vi "Adam_Ch_Input_Output_ASYNC.vi"(4 "Client Name":string, 6 "Previous Scan Value":dbl format="%.2f", 7 "Value to Output":dbl format="%.2f", 8 "Ch values":dbl[](array[numeric]) format="%.2f", 9 "Scan Period":dbl format="%.2f", 10 "Ch Description":T1={"Ch Name"="", "Type"="", "Function"=enum."Analogue Input", "Ch State"=enum."On", "Calibration type"="", "A"=0.0, "B"=0.0, "C"=0.0, "D"=0.0, "Comments"="", "Address"={"Main"=0, "Ch."=0, "Sub"=0, "Port Name"=""}, "String"="", "Duty"=65535} {"Duty" format="%016b"; "D" format="%#_5g"; "C" format="%#_5g"; "B" format="%#_5g"; "A" format="%#_5g"}, 11 "Ch names":string[](array[string])) -> (1 "Calibrated units":dbl format="%.2f", 3 "Scan comment":string)   [LabVIEW 2020]
uses:
  ADAM Client/Sub VIs/ADAM Controls/Ch_description_ADAM.ctl
  ADAM Client/Sub VIs/ADAM Controls/Module_type_ADAM.ctl
  ADAM Client/Sub VIs/ADAM Controls/Function_ADAM.ctl
  ADAM Client/Sub VIs/ADAM Controls/Channel_State.ctl
  ADAM Client/Sub VIs/ADAM Controls/Calib_type_ADAM.ctl
  ADAM Client/Sub VIs/ADAM Controls/Address.ctl
  Anemometry/Anemometry Sub Vis/Controls/Serveds.ctl
  ADAM Client/Sub VIs/ADAM Controls/Update_scan_value.ctl
  ADAM_Global.vi
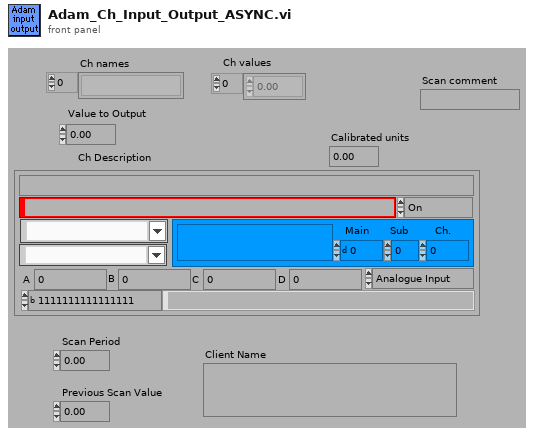
[diagram p1: front panel]
types:
  T1 = typedef "Ch_description_ADAM.ctl" = cluster{"Ch Name":string, "Type":T2, "Function":T3, "Ch State":T4, "Calibration type":T5, "A":dbl, "B":dbl, "C":dbl, "D":dbl, "Comments":string, "Address":T6, "String":string, "Duty":u16}
  T2 = typedef "Module_type_ADAM.ctl" = string
  T3 = typedef "Function_ADAM.ctl" = enum16{"Analogue Input", "Digital Input", "Event counter", "Event rate", "Analogue Output", "Digital Output", "Relay Output"}
  T4 = typedef "Channel_State.ctl" = enum16{"On", "Off", "Always On", "Always Off"}
  T5 = typedef "Calib_type_ADAM.ctl" = string
  T6 = typedef "Address.ctl" = cluster{"Main":i32, "Ch.":i32, "Sub":i32, "Port Name":string}
  T7 = enum16{"Channel Unshared", "Channel Shared by Rig", "Channel Shared by Group"}
  T8 = typedef "Serveds.ctl" = enum16{"Read Global", "Load Global From File"}
  T9 = enum16{"Append to Global", "Read Global then Clear"}
  T10 = typedef "Update_scan_value.ctl" = cluster{"Channel Name":string, "New Value":dbl}
  T11 = typedef "Server_Control.ctl" = cluster{"Channel Name to control":string, "Channel sharing":enum16{"Channel Unshared", "Channel Shared by Rig", "Channel Shared by Group"}, "Default Value":dbl, "Client Array":string[], "Time Stamp":timestamp, "Do Not Reset":bool}
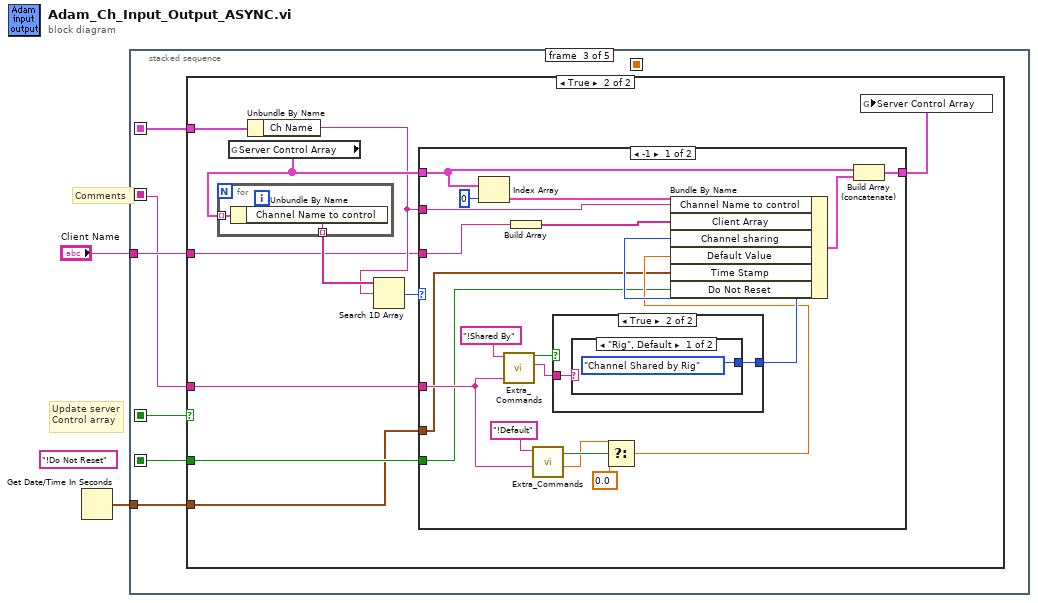
[diagram p0: block diagram]
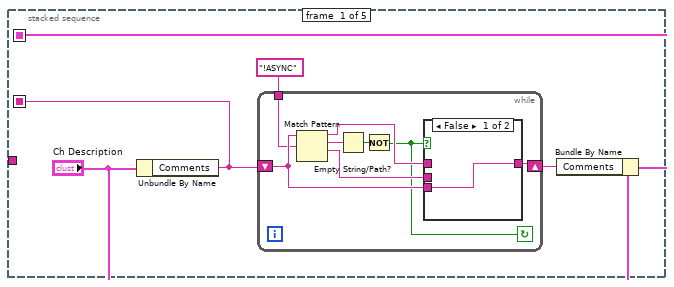
[diagram p2: hidden frame]
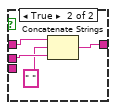
[diagram p3: hidden frame]
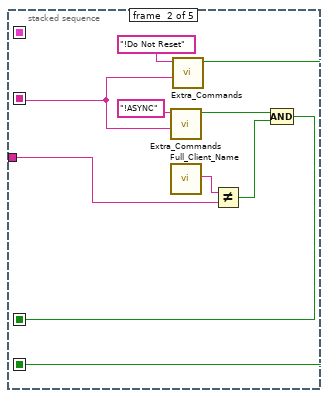
[diagram p4: hidden frame]
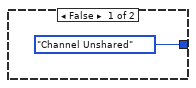
[diagram p6: hidden frame]
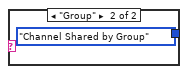
[diagram p7: hidden frame]
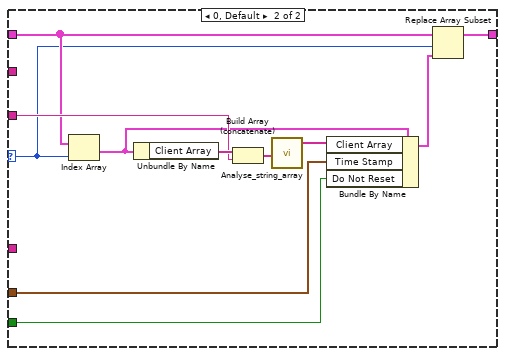
[diagram p8: hidden frame]
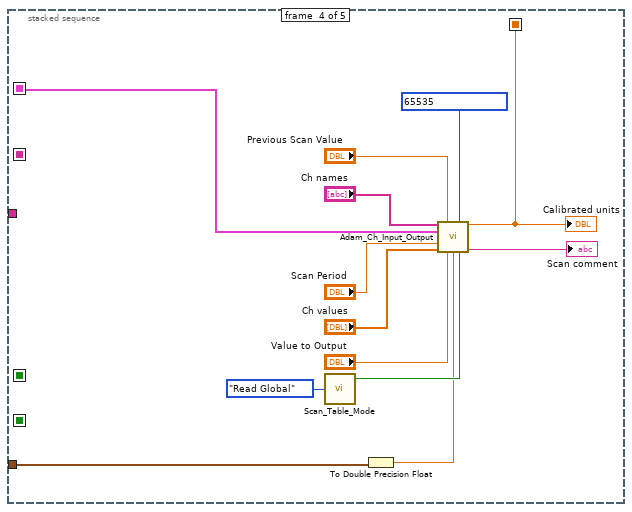
[diagram p9: hidden frame]
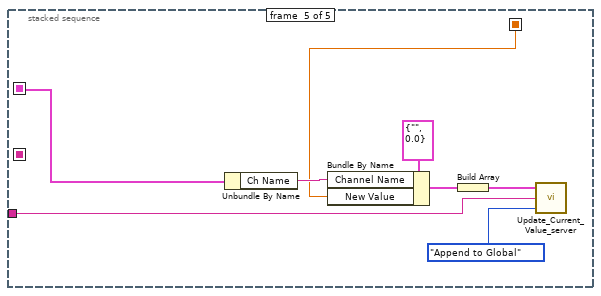
[diagram p10: hidden frame]
diagram:
  (unwired) "!Do Not Reset" ("String to match")
  # "Update server\nControl array"
  # "Comments"
  n1 = Get Date/Time In Seconds() -> (seconds since 1Jan1904=w1:timestamp)
  n2 = stacked-sequence {
    seq-local: [w6 _ _ _ _] -> [_ _ w32 w96 w104]
    seq-local: [_ _ _ w91 _] -> [_ _ _ _ w100]
    seq-local: [w5 _ _ _ _] -> [_ w27 w34 _ _]
    seq-local: [_ w22 _ _ _] -> [_ _ w33 _ _]
    seq-local: [_ w21 _ _ _] -> [_ _ w31 _ _]
    tunnel: "Client Name" -> [_ w24 w35 _ w97]
    tunnel: w1 -> [_ _ w30 w84 _]
    frame #0 {
      n3 = Unbundle By Name("Ch Description") -> ("Comments"=w5:string)
      n4 = while {
        shift-left: w5 -> [w12]
        shift-right: [w13] -> w7
        tunnel: "!ASYNC" ("String to match") -> [w8]
        stop <- w9 continue-if-true
        n5 = Match Pattern(string=w12, regular expression=w8) -> (before substring=w11:string, match substring=w15:string, after substring=w10:string)  [unwired: 2 out]
        n6 = Empty String/Path?(string/path=w15) -> (empty?=w14:bool)
        n7 = Not(x=w14) -> (.not. x?=w9:bool)
        n8 = case shown="False" w9 {
          tunnel: [w16 w19] -> w13
          tunnel: w12 -> [w16 _]
          tunnel: w11 -> [_ w20]
          tunnel: w10 -> [_ w18]
          frame False {
          }
          frame True {
            n9 = Concatenate Strings(w20, " " ("After  Matched string"), w18) -> (w19:string)
          }
        }
      }
      n10 = Bundle By Name(cluster="Ch Description", "Comments"=w7) -> (w6:T1)
    }
    frame #1 {
      n11 = call "Extra_Commands.vi"("String to Search"=w27, "Command"="!ASYNC" ("String to match")) -> ("Command Found"=w26:bool)  [unwired: 1 in, 4 out]
      n12 = call "Full_Client_Name.vi"() -> ("Client Name"=w25:string)
      n13 = call "Extra_Commands.vi"("String to Search"=w27, "Command"="!Do Not Reset" ("String to match")) -> ("Command Found"=w21:bool)  [unwired: 1 in, 4 out]
      n14 = Not Equal?(x=w25, y=w24) -> (x != y?=w23:bool)
      n15 = Compound Arithmetic op=AND(w26, w23) -> (w22:bool)
    }
    frame #2 {
      n16 = case shown="True" w33 {
        tunnel: w34 -> [_ w44]
        tunnel: w35 -> [_ w38]
        tunnel: w32 -> [_ w45]
        tunnel: w31 -> [_ w37]
        tunnel: w30 -> [_ w36]
        frame False {
        }
        frame True {
          n17 = global read "ADAM_Global.vi" "Server Control Array"() -> (w42:T11[])
          n18 = for {
            tunnel: w42 -> [w47] mode=indexing
            tunnel: [w46] -> w41 mode=indexing
            n19 = Unbundle By Name(w47) -> ("Channel Name to control"=w46:string)
          }
          n20 = Unbundle By Name(w45) -> ("Ch Name"=w39:string)
          n21 = Search 1D Array(1D array=w41, element=w39) -> (index of element=w40:i32)  [unwired: 1 out]
          n22 = case shown="-1" w40 {
            selector: w40 -> [_ w73]
            tunnel: [w50 w83] -> w43
            tunnel: w38 -> [w54 w81]
            tunnel: w42 -> [w52 w76]
            tunnel: w39 -> [w55 _]
            tunnel: w44 -> [w53 _]
            tunnel: w36 -> [w49 w75]
            tunnel: w37 -> [w48 w74]
            frame -1 {
              n23 = Index Array(array=w52, index=0 ("Index")) -> (element=w56:T11)
              n24 = call "Extra_Commands.vi"("String to Search"=w53, "Command"="!Shared By") -> ("String Value"=w66:string, "Command Found"=w65:bool)  [unwired: 1 in, 3 out]
              n25 = Build Array(w54) -> (w58:string[])
              n26 = call "Extra_Commands.vi"("String to Search"=w53, "Command"="!Default") -> ("Numeric Value"=w61:dbl, "Command Found"=w62:bool)  [unwired: 1 in, 3 out]
              n27 = case shown="True" w65 {
                tunnel: w66 -> [_ w70]
                tunnel: [T7."Channel Unshared" ("Bundle Element") w69] -> w64
                frame False {
                }
                frame True {
                  n28 = case shown="\"Rig\", Default" w70 {
                    tunnel: [T7."Channel Shared by Rig" ("Bundle Element") T7."Channel Shared by Group" ("Bundle Element")] -> w69
                    frame "Rig", Default {
                    }
                    frame "Group" {
                    }
                  }
                }
              }
              n29 = Select(t=w61, s=w62, f=0.0) -> (s? t:f=w59:dbl)
              n30 = Bundle By Name(cluster=w56, "Channel Name to control"=w55, "Client Array"=w58, "Channel sharing"=w64, "Default Value"=w59, "Time Stamp"=w49, "Do Not Reset"=w48) -> (w51:T11)
              n31 = Build Array (concatenate)(w52, w51) -> (w50:T11[])
            }
            frame 0, Default {
              n32 = Index Array(array=w76, index=w73) -> (element=w79:T11)
              n33 = Unbundle By Name(w79) -> ("Client Array"=w82:string[])
              n34 = Build Array (concatenate)(w82, w81) -> (w80:string[])
              n35 = call "Analyse_string_array.vi"("String array"=w80) -> ("Unique strings"=w78:string[])  [unwired: 2 out]
              n36 = Bundle By Name(cluster=w79, "Client Array"=w78, "Time Stamp"=w75, "Do Not Reset"=w74) -> (w77:T11)
              n37 = Replace Array Subset(array=w76, new element=w77, index=w73) -> (w83:T11[])
            }
          }
          n38 = global write "ADAM_Global.vi" "Server Control Array"(w43) -> ()
        }
      }
    }
    frame #3 {
      n39 = call "Scan_Table_Mode.vi"("Mode"=Serveds."Read Global") -> ("Simulate Mode ?"=w86:bool)  [unwired: 2 out]
      n40 = To Double Precision Float(number=w84) -> (double precision float=w85:dbl)
      n41 = call "Adam_Ch_Input_Output.vi"("Ch names"="Ch names", "Previous Scan Value"="Previous Scan Value", "Duty No"=u16 65535, "Ch Description"=w96, "Scan Period"="Scan Period", "Ch values"="Ch values", "Value to Output"="Value to Output", "Current Time (sec)"=w85, "Simulate"=w86) -> ("Calibrated units"=w91:dbl, "Scan comment"=→"Scan comment":string)  [unwired: 3 in, 2 out]
      "Calibrated units" <- w91
    }
    frame #4 {
      n42 = Unbundle By Name(w104) -> ("Ch Name"=w102:string)
      n43 = Bundle By Name(cluster=T10 {"Channel Name"="", "New Value"=0.0} ("Update Scan Value Cluster"), "Channel Name"=w102, "New Value"=w100) -> (w101:T10)
      n44 = Build Array(w101) -> (w99:T10[])
      n45 = call "Update_Current_Value_server.vi"("Mode"=T9."Append to Global", "Client HD name"=w97, "Update array in"=w99) -> ()  [unwired: 1 out]
    }
  }
